vi "Source_Voltage.vi"(4 "Source Delay (Sec)":dbl=0.1 format="%.3p", 6 "Current Limit Range":dbl=0.01 format="%.3p", 7 "Current Limit":dbl=0.01 format="%.3p", 8 "error in (no error)":errorcluster, 9 "Voltage Level Range":dbl=6.0 format="%.5p", 10 "Voltage Level":dbl=2.0 format="%.5p", 11 "niDCPower in":refnum<class "niDCPower.lvclass">) -> (0 "error out":errorcluster, 3 "niDCPower out":refnum<class "niDCPower.lvclass">)   [LabVIEW 2021, in "niDCPower.lvclass"]
uses:
  niDCPower.lvclass
  <instrlib>/niDCPower/nidcpower.llb/niDCPower Source Mode.ctl
  <instrlib>/niDCPower/nidcpower.llb/niDCPower Output Function.ctl
  niDCPower.lvclass/niDCPower.ctl
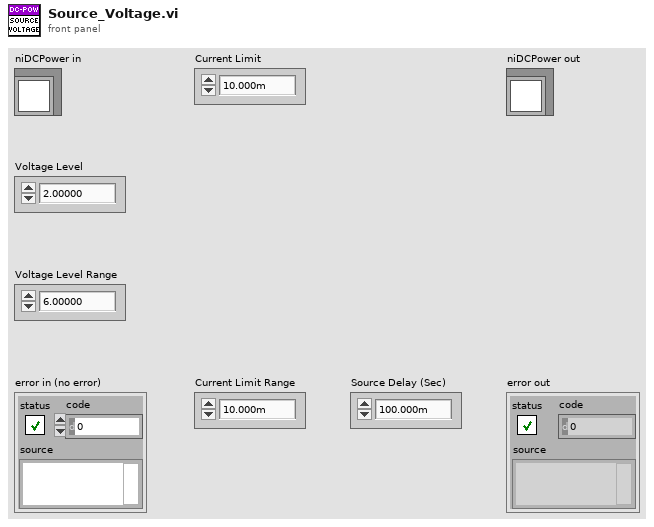
[diagram p1: front panel]
types:
  T1 = typedef "niDCPower Output Function.ctl" = i32
  T2 = typedef "niDCPower Source Mode.ctl" = i32
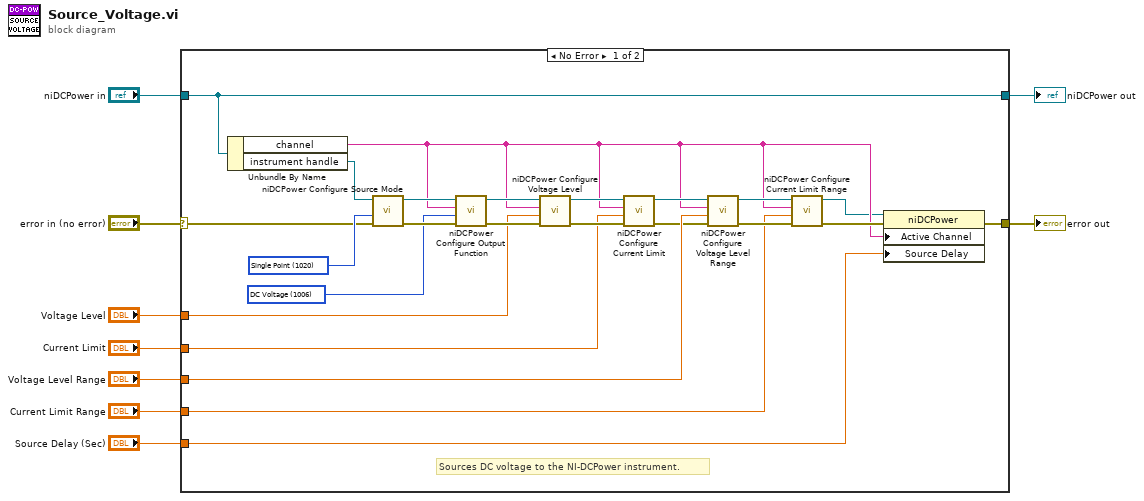
[diagram p0: block diagram]
diagram:
  n1 = case shown="No Error" "error in (no error)" {
    selector: "error in (no error)" -> [w26 w35]
    tunnel: "niDCPower in" -> [w10 w34]
    tunnel: "Voltage Level" -> [w25 _]
    tunnel: "Voltage Level Range" -> [w24 _]
    tunnel: "Source Delay (Sec)" -> [w23 _]
    tunnel: [w22 w35] -> w4
    tunnel: "Current Limit" -> [w19 _]
    tunnel: "Current Limit Range" -> [w12 _]
    tunnel: [w10 w34] -> w1
    frame No Error {
      w28 = T1 1006 items=["DC Voltage"=1006, "DC Current"=1007, "Pulse Voltage"=1049, "Pulse Current"=1050] ("output function")
      w29 = T2 1020 items=["Single Point"=1020, "Sequence"=1021] ("source mode")
      # "Sources DC voltage to the NI-DCPower instrument."
      n2 = Unbundle By Name(w10) -> ("channel"=w13:string, "instrument handle"=w30:refnum<k15>)
      n3 = call <instrlib>:"niDCPower Configure Source Mode.vi"("error in (no error)"=w26, "source mode"=w29, "instrument handle"=w30) -> ("error out"=w32:errorcluster, "instrument handle out"=w33:refnum<k15>)  [unwired: 7 out]
      n4 = call <instrlib>:"niDCPower Configure Output Function.vi"("error in (no error)"=w32, "output function"=w28, "channel name"=w13, "instrument handle"=w33) -> ("error out"=w31:errorcluster, "instrument handle out"=w27:refnum<k15>)  [unwired: 6 out]
      n5 = call <instrlib>:"niDCPower Configure Voltage Level.vi"("error in (no error)"=w31, "voltage level"=w25, "channel name"=w13, "instrument handle"=w27) -> ("error out"=w21:errorcluster, "instrument handle out"=w14:refnum<k15>)  [unwired: 6 out]
      n6 = call <instrlib>:"niDCPower Configure Current Limit.vi"("error in (no error)"=w21, "current limit"=w19, "channel name"=w13, "instrument handle"=w14) -> ("error out"=w20:errorcluster, "instrument handle out"=w15:refnum<k15>)  [unwired: 1 in, 5 out]
      n7 = call <instrlib>:"niDCPower Configure Voltage Level Range.vi"("error in (no error)"=w20, "voltage level range"=w24, "channel name"=w13, "instrument handle"=w15) -> ("error out"=w18:errorcluster, "instrument handle out"=w16:refnum<k15>)  [unwired: 6 out]
      n8 = call <instrlib>:"niDCPower Configure Current Limit Range.vi"("error in (no error)"=w18, "current limit range"=w12, "channel name"=w13, "instrument handle"=w16) -> ("error out"=w17:errorcluster, "instrument handle out"=w11:refnum<k15>)  [unwired: 6 out]
      n9 = property class="niDCPower"(reference=w11, error in=w17, "Active Channel"=w13, "Source Delay"=w23) -> (error out=w22:errorcluster)  [unwired: 1 out]
    }
    frame Error {
    }
  }
  "error out" <- w4
  "niDCPower out" <- w1
